vi "Read Depth Scale.vi"(8 "error in (no error)":errorcluster, 11 "Realsense Cam File Wrapper in":refnum<class "Realsense Cam File Wrapper.lvclass">) -> (0 "error out":errorcluster, 2 "Depth Scale":dbl, 3 "Realsense Cam File Wrapper out":refnum<class "Realsense Cam File Wrapper.lvclass">)   [LabVIEW 2018, in "Realsense Cam File Wrapper.lvclass"]
uses:
  Realsense Cam File Wrapper.lvclass
  Realsense Cam File Wrapper.lvclass/Realsense Cam File Wrapper.ctl
  Realsense Cam/Realsense Cam.lvclass
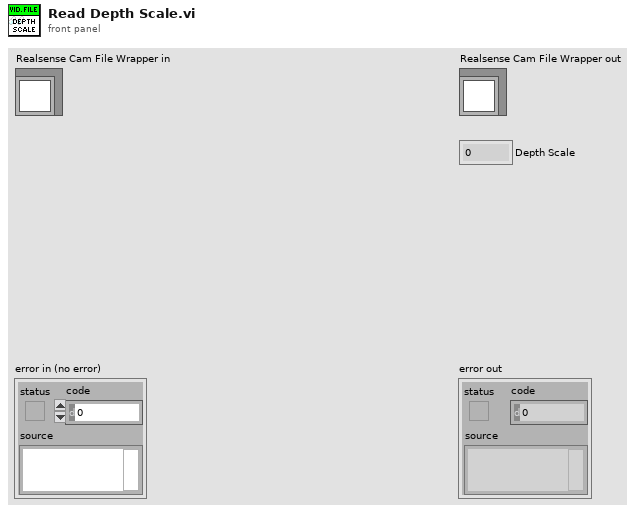
[diagram p1: front panel]
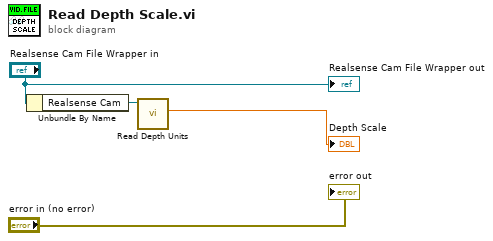
[diagram p0: block diagram]
diagram:
  n1 = Unbundle By Name("Realsense Cam File Wrapper in") -> ("Realsense Cam"=w4:refnum<class "Realsense Cam.lvclass">)
  n2 = call-dynamic "Read Depth Units.vi"("Realsense Cam in"=w4) -> ("Depth Units"=→"Depth Scale":dbl)  [unwired: 8 in, 2 out]
  "error out" <- "error in (no error)"
  "Realsense Cam File Wrapper out" <- "Realsense Cam File Wrapper in"
